vi "StepMotorStateMachine.vi"() -> ()   [LabVIEW 2015]
panel:
  out "Descripción de Elementos":string="Diagrama Fasorial donde se\nmuestra el ángulo de la vuelta\nrealizada por el motor a pasos"
  in  "y":i32=360
  out "Angulo":i32
  out "Diagrama Fasorial":picture
  out "Gauge":dbl(knob)=360.0 scale=0.0..360.0
  out "Contador de\nVueltas":i32
  in  "Direccion de Giro":bool=TRUE
  in  "stop":bool
  out "Control del Motor":bool[](array[boolean])=[FALSE, TRUE, TRUE, FALSE]
  out "Estado Booleano":bool[](array[boolean])=[FALSE, TRUE, TRUE, FALSE, FALSE, FALSE, FALSE, FALSE, FALSE, FALSE, FALSE, FALSE, FALSE, FALSE, FALSE, FALSE, FALSE, FALSE, FALSE, FALSE, FALSE, FALSE, FALSE, FALSE, FALSE, FALSE, FALSE, FALSE, FALSE, FALSE, FALSE, FALSE]
  out "Estado":u8=6
  in  "Control de\nVelocidad":u32(knob) scale=0.0..300.0
  # "Serrano Bermúdez Luis Esteban"
  # "6/Abril/2019"
  # "Control de Velocidad y Seguimiento de un Motor a pasos"
  # "Descripción: A partir de una tarjeta DAQ configurada para\n                    generar y adquirir señales mueve un motor a pasos\n                    que se mostrará en un diagrama fasorial así en un\n                    medidor de brujula (Gauge) de 360° la posicion y el\n                    número de vueltas realizadas"
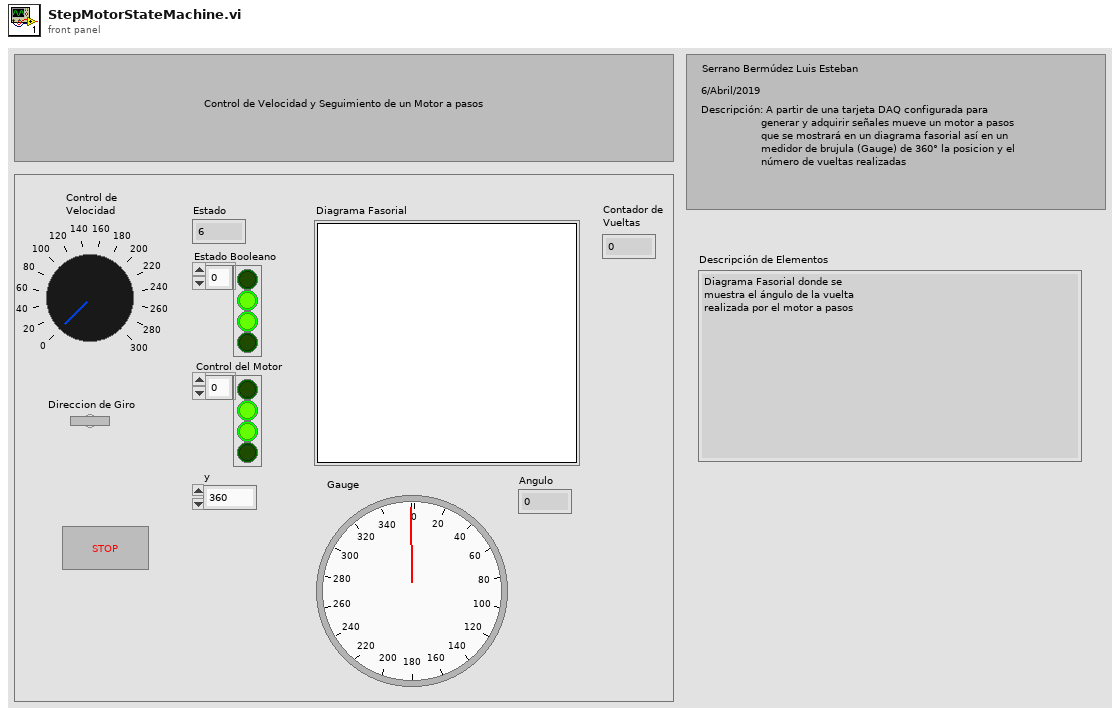
[diagram p1: front panel]
types:
  T1 = typedef "LVBoundsTypeDef.ctl" = cluster{"Width":u32, "Height":u32}
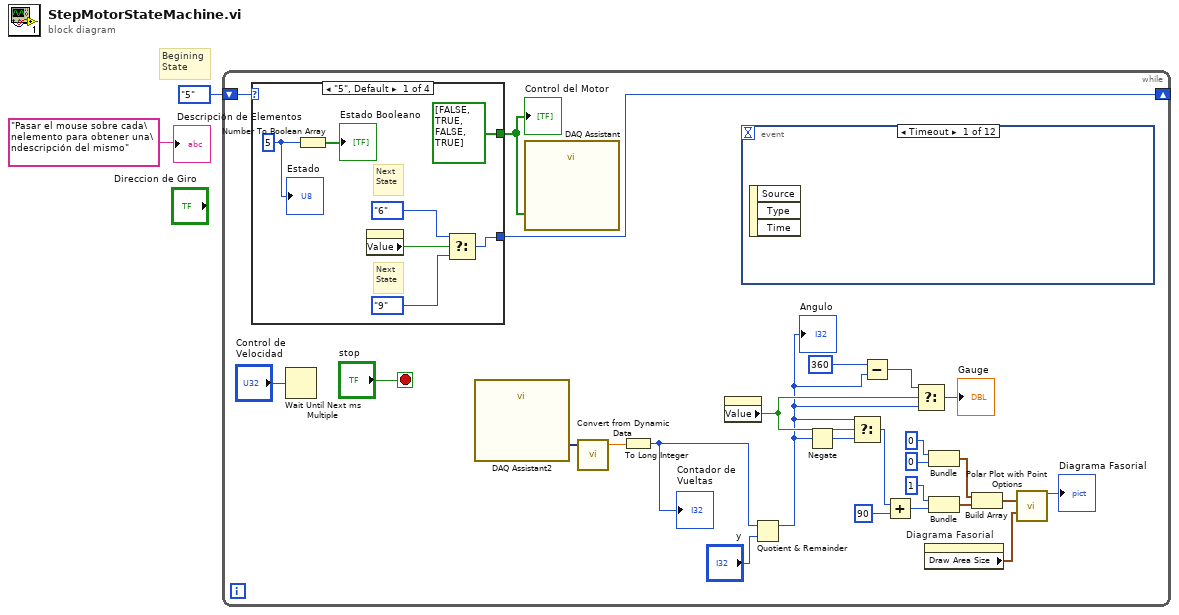
[diagram p0: block diagram]
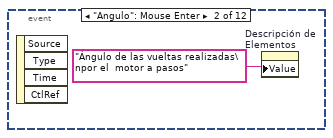
[diagram p2: hidden frame]
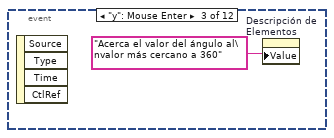
[diagram p3: hidden frame]
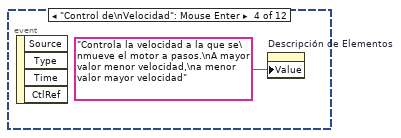
[diagram p4: hidden frame]
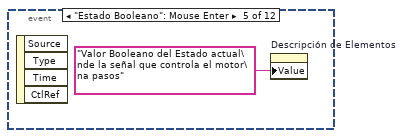
[diagram p5: hidden frame]
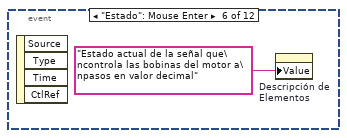
[diagram p6: hidden frame]
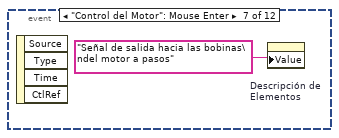
[diagram p7: hidden frame]
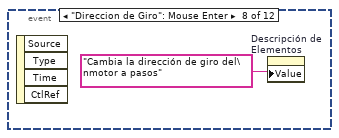
[diagram p8: hidden frame]
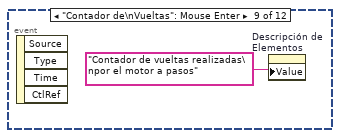
[diagram p9: hidden frame]
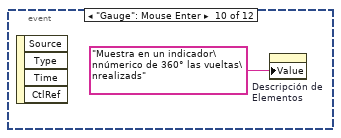
[diagram p10: hidden frame]
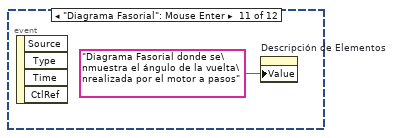
[diagram p11: hidden frame]
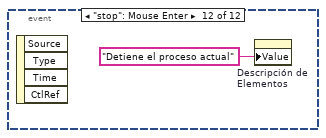
[diagram p12: hidden frame]
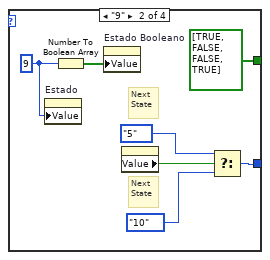
[diagram p13: hidden frame]
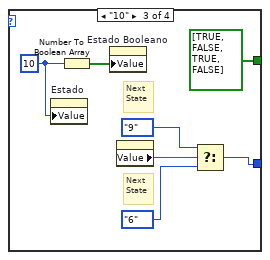
[diagram p14: hidden frame]
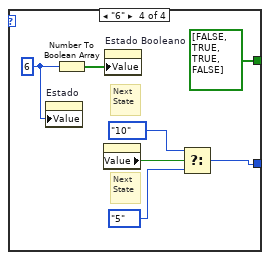
[diagram p15: hidden frame]
diagram:
  # "Begining\nState"
  n1 = while {
    shift-right: [w27] -> _
    shift-left: enum16{"5", "9", "10", "6"}."5" -> [w28]
    stop <- "stop" stop-if-true
    n2 = case shown="\"5\", Default" w28 {
      tunnel: [bool[] [FALSE, TRUE, FALSE, TRUE] bool[] [TRUE, FALSE, FALSE, TRUE] bool[] [TRUE, FALSE, TRUE, FALSE] bool[] [FALSE, TRUE, TRUE, FALSE]] -> w25
      tunnel: [w40 w47 w54 w61] -> w27
      frame "5", Default {
        w46 = 5
        # "Next\nState"
        # "Next\nState"
        n3 = Number To Boolean Array(number=w46) -> (Boolean array=→"Estado Booleano":bool[])
        n4 = property on="Direccion de Giro" class="Bool (strict)"() -> ("Value"=w41:bool)  [unwired: 2 in, 2 out]
        n5 = Select(t=enum16{"5", "9", "10", "6"}."6", s=w41, f=enum16{"5", "9", "10", "6"}."9") -> (s? t:f=w40:enum16{"5", "9", "10", "6"})
        "Estado" <- w46
      }
      frame "9" {
        w52 = 9
        # "Next\nState"
        # "Next\nState"
        n6 = property on="Estado" class="DigNum (strict)"("Value"=w52) -> ()  [unwired: 2 in, 2 out]
        n7 = Number To Boolean Array(number=w52) -> (Boolean array=w53:bool[])
        n8 = property on="Estado Booleano" class="Arr (strict)"("Value"=w53) -> ()  [unwired: 2 in, 2 out]
        n9 = property on="Direccion de Giro" class="Bool (strict)"() -> ("Value"=w50:bool)  [unwired: 2 in, 2 out]
        n10 = Select(t=enum16{"5", "9", "10", "6"}."5", s=w50, f=enum16{"5", "9", "10", "6"}."10") -> (s? t:f=w47:enum16{"5", "9", "10", "6"})
      }
      frame "10" {
        w59 = 10
        # "Next\nState"
        # "Next\nState"
        n11 = property on="Estado" class="DigNum (strict)"("Value"=w59) -> ()  [unwired: 2 in, 2 out]
        n12 = Number To Boolean Array(number=w59) -> (Boolean array=w60:bool[])
        n13 = property on="Estado Booleano" class="Arr (strict)"("Value"=w60) -> ()  [unwired: 2 in, 2 out]
        n14 = property on="Direccion de Giro" class="Bool (strict)"() -> ("Value"=w57:bool)  [unwired: 2 in, 2 out]
        n15 = Select(t=enum16{"5", "9", "10", "6"}."9", s=w57, f=enum16{"5", "9", "10", "6"}."6") -> (s? t:f=w54:enum16{"5", "9", "10", "6"})
      }
      frame "6" {
        w66 = 6
        # "Next\nState"
        # "Next\nState"
        n16 = property on="Estado" class="DigNum (strict)"("Value"=w66) -> ()  [unwired: 2 in, 2 out]
        n17 = Number To Boolean Array(number=w66) -> (Boolean array=w67:bool[])
        n18 = property on="Direccion de Giro" class="Bool (strict)"() -> ("Value"=w64:bool)  [unwired: 2 in, 2 out]
        n19 = property on="Estado Booleano" class="Arr (strict)"("Value"=w67) -> ()  [unwired: 2 in, 2 out]
        n20 = Select(t=enum16{"5", "9", "10", "6"}."10", s=w64, f=enum16{"5", "9", "10", "6"}."5") -> (s? t:f=w61:enum16{"5", "9", "10", "6"})
      }
    }
    "Control del Motor" <- w25
    n21 = Wait Until Next ms Multiple(millisecond multiple="Control de\nVelocidad") -> ()  [unwired: 1 out]
    n22 = call "DAQ Assistant2"() -> ("data"=w12:dynamicdata)  [unwired: 16 in, 3 out]
    n23 = call "DAQ Assistant"("data"=w25) -> ()  [unwired: 17 in, 2 out]
    n24 = call "Convert from Dynamic Data"("Dynamic Data Type"=w12) -> ("Scalar"=w11:dbl)  [unwired: 3 in]
    n25 = To Long Integer(number=w11) -> (32bit integer=w10:i32)
    "Contador de\nVueltas" <- w10
    n26 = property on="Direccion de Giro" class="Bool (strict)"() -> ("Value"=w6:bool)  [unwired: 2 in, 2 out]
    n27 = event shown="[0] Timeout" {
      selector: _ -> [_ _ _ _ _ _ _ _ _ _ _ _]
      dyn-events: _ -> [_ _ _ _ _ _ _ _ _ _ _ _]
      timeout: _ -> [_ _ _ _ _ _ _ _ _ _ _ _]
      event Timeout {
        n28 = event-data() -> ()  [unwired: 1 in, 3 out]
      }
      event "Angulo": Mouse Enter {
        n29 = event-data() -> ()  [unwired: 1 in, 4 out]
        n30 = property on="Descripción de Elementos" class="Str"("Value"="Ángulo de las vueltas realizadas\npor el  motor a pasos" ("String")) -> ()  [unwired: 2 in, 2 out]
      }
      event "y": Mouse Enter {
        n31 = event-data() -> ()  [unwired: 1 in, 4 out]
        n32 = property on="Descripción de Elementos" class="Str"("Value"="Acerca el valor del ángulo al\nvalor más cercano a 360" ("String")) -> ()  [unwired: 2 in, 2 out]
      }
      event "Control de\nVelocidad": Mouse Enter {
        n33 = event-data() -> ()  [unwired: 1 in, 4 out]
        n34 = property on="Descripción de Elementos" class="Str"("Value"="Controla la velocidad a la que se\nmueve el motor a pasos.\nA mayor valor menor velocidad,\na menor valor mayor velocidad" ("String")) -> ()  [unwired: 2 in, 2 out]
      }
      event "Estado Booleano": Mouse Enter {
        n35 = event-data() -> ()  [unwired: 1 in, 4 out]
        n36 = property on="Descripción de Elementos" class="Str"("Value"="Valor Booleano del Estado actual\nde la señal que controla el motor\na pasos" ("String")) -> ()  [unwired: 2 in, 2 out]
      }
      event "Estado": Mouse Enter {
        n37 = event-data() -> ()  [unwired: 1 in, 4 out]
        n38 = property on="Descripción de Elementos" class="Str"("Value"="Estado actual de la señal que\ncontrola las bobinas del motor a\npasos en valor decimal" ("String")) -> ()  [unwired: 2 in, 2 out]
      }
      event "Control del Motor": Mouse Enter {
        n39 = event-data() -> ()  [unwired: 1 in, 4 out]
        n40 = property on="Descripción de Elementos" class="Str"("Value"="Señal de salida hacia las bobinas\ndel motor a pasos" ("String")) -> ()  [unwired: 2 in, 2 out]
      }
      event "Direccion de Giro": Mouse Enter {
        n41 = event-data() -> ()  [unwired: 1 in, 4 out]
        n42 = property on="Descripción de Elementos" class="Str"("Value"="Cambia la dirección de giro del\nmotor a pasos" ("String")) -> ()  [unwired: 2 in, 2 out]
      }
      event "Contador de\nVueltas": Mouse Enter {
        n43 = event-data() -> ()  [unwired: 1 in, 4 out]
        n44 = property on="Descripción de Elementos" class="Str"("Value"="Contador de vueltas realizadas\npor el motor a pasos" ("String")) -> ()  [unwired: 2 in, 2 out]
      }
      event "Gauge": Mouse Enter {
        n45 = event-data() -> ()  [unwired: 1 in, 4 out]
        n46 = property on="Descripción de Elementos" class="Str"("Value"="Muestra en un indicador\nnúmerico de 360° las vueltas\nrealizads" ("String")) -> ()  [unwired: 2 in, 2 out]
      }
      event "Diagrama Fasorial": Mouse Enter {
        n47 = event-data() -> ()  [unwired: 1 in, 4 out]
        n48 = property on="Descripción de Elementos" class="Str"("Value"="Diagrama Fasorial donde se\nmuestra el ángulo de la vuelta\nrealizada por el motor a pasos" ("String")) -> ()  [unwired: 2 in, 2 out]
      }
      event "stop": Mouse Enter {
        n49 = event-data() -> ()  [unwired: 1 in, 4 out]
        n50 = property on="Descripción de Elementos" class="Str"("Value"="Detiene el proceso actual" ("String")) -> ()  [unwired: 2 in, 2 out]
      }
    }
    n51 = Quotient & Remainder(x=w10, y="y") -> (x-y*floor(x/y)=w3:i32)  [unwired: 1 out]
    "Angulo" <- w3
    n52 = Negate(x=w3) -> (-x=w8:i32)
    n53 = Select(t=w3, s=w6, f=w8) -> (s? t:f=w9:i32)
    n54 = Subtract(x=360, y=w3) -> (x-y=w4:i32)
    n55 = Add(x=w9, y=90) -> (x+y=w13:i32)
    n56 = Select(t=w4, s=w6, f=w3) -> (s? t:f=→"Gauge":i32)
    n57 = property on="Diagrama Fasorial" class="Pict"() -> ("Draw Area Size"=w21:T1)  [unwired: 2 in, 2 out]
    n58 = Bundle(0, 0) -> (w18:cluster{i32, i32})  [unwired: 1 in]
    n59 = Bundle(1, w13) -> (w15:cluster{i32, i32})  [unwired: 1 in]
    n60 = Build Array(w18, w15) -> (w17:cluster{i32, i32}[])
    n61 = call <vilib>:"Polar Plot with Point Options.vi"("data array [mag, phase (deg)]"=w17, "dimensions (w,h)"=w21) -> ("new picture"=→"Diagrama Fasorial":picture)  [unwired: 13 in]
  }
  "Descripción de Elementos" <- "Pasar el mouse sobre cada\nelemento para obtener una\ndescripción del mismo"
